vi "DAQ_Static Dig Gen Initialize.vi"(0 "Physical Channels":tag, 7 "Global Channels":refnum<k21>, 11 "error in":errorcluster) -> (4 "DAQmx Task Out":refnum<k21>, 15 "error out":errorcluster)   [LabVIEW 2021, in "DAQ_Static Digital State Generation.lvlib"]
doc: "Initialize Digital Output channels and obtains a DAQmx task\n\nProvide either Physical channel or Global Channel\nIf both physical and Global channels are provided, Global Channels will take precedence\n\n<B>Note:</B> This Library supports only digital line in the physical/global channel. Port is not supported in this library and returns an error. User can either use <B>Dynamic Digital Pattern Measurement Library</B> to support port based inputs or specify the ports in line based format (Ex: <B>DIO/port0/line0:31</B>) with the current library."
uses:
  DAQ_Static Digital State Generation.lvlib
  <vilib>/DAQmx/create/channels.llb/DAQmx Create Channel (DO-Digital Output).vi
panel:
  # "Inputs"
  # "Outputs"
  # "Overview:\nThis VI initializes Digital output channels for static digital generation and provides the DAQmx Task Out\n\nHardware Requirement: A compatible PXI, PCIe, USB, cDAQ or Testscale device\n\nSoftware Requirement: NI DAQmx 2022Q4 or later\n\nInstructions:\n1. Enter physical channel in which Static Digital State Generation has to be done in Physical Channels control. (Or) Enter Global channels to use it instead of initiating a new task. User must configure only one input. If both are provided, Global Channels will take precedence..\n2. Get the Digital Generation task from DAQmx Task Out which stores the reference to the virtual digital output channels.\n\nNotes: \n1. User can use the DAQmx Task on other VI in this library to configure and initiate digital state generation task.\n2. This Library supports only digital line in the physical/global channel. Port is not supported in this library and returns an error. User can either use Dynamic Digital Pattern Measurement Library to support port-based inputs or specify the ports in line based format (Ex: DIO/port0/line0:31) with the current library."
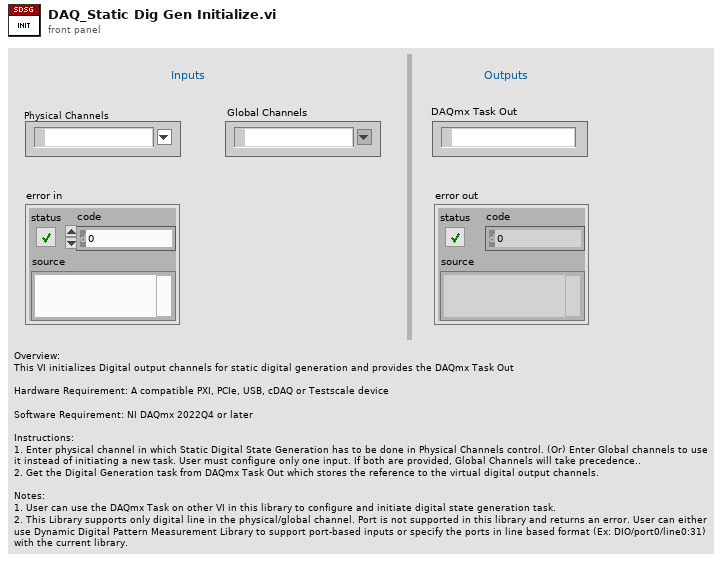
[diagram p1: front panel]
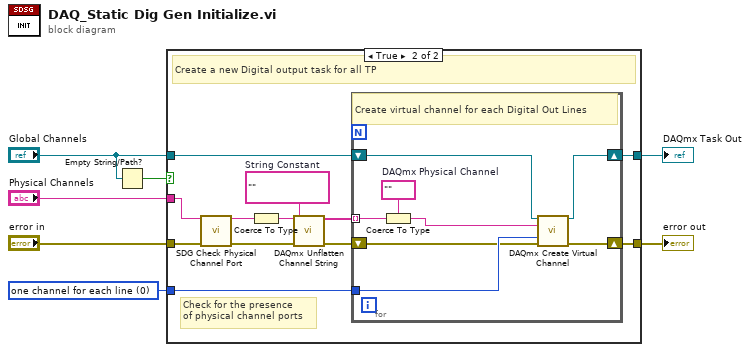
[diagram p0: block diagram]
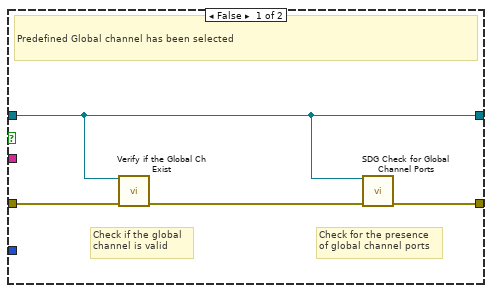
[diagram p2: hidden frame]
diagram:
  w3 = 0 items=["one channel for each line", "one channel for all lines"] ("line grouping")
  n1 = Empty String/Path?(string/path="Global Channels") -> (empty?=w4:bool)
  n2 = case shown="True" w4 {
    tunnel: "Physical Channels" -> [_ w16]
    tunnel: "Global Channels" -> [w11 w23]
    tunnel: [w11 w21] -> w1
    tunnel: "error in" -> [w10 w17]
    tunnel: [w8 w20] -> w2
    tunnel: w3 -> [_ w22]
    frame False {
      # "Check for the presence\nof global channel ports"
      # "Check if the global\nchannel is valid"
      # "Predefined Global channel has been selected"
      n3 = call "Verify if the Global Ch Exist.vi"("Global Channels"=w11, "error in (no error)"=w10) -> ("error out"=w9:errorcluster)  [unwired: 13 in]
      n4 = call "SDG Check for Global Channel Ports.vi"("Global Channel In"=w11, "error in (no error)"=w9) -> ("error out"=w8:errorcluster)  [unwired: 12 in, 1 out]
    }
    frame True {
      w15 = ""  # String Constant
      # "Check for the presence \nof physical channel ports"
      # "Create a new Digital output task for all TP"
      n5 = call "SDG Check Physical Channel Port.vi"("Physical Channel In"=w16, "error in (no error)"=w17) -> ("Physical Channel Out"=w14:tag, "error out"=w12:errorcluster)  [unwired: 12 in]
      n6 = Coerce To Type(0:w14, 1:w15) -> (2:w13:string)
      n7 = call <vilib>:"DAQmx Unflatten Channel String.vi"("names in"=w13, "error in"=w12) -> ("names out"=w19:string[], "error out"=w18:errorcluster)  [unwired: 12 in]
      n8 = for {
        shift-right: [w30] -> w21
        shift-left: w23 -> [w31]
        shift-right: [w29] -> w20
        shift-left: w18 -> [w27]
        tunnel: w19 -> [w26] mode=indexing
        tunnel: w22 -> [w28]
        w25 = tag ""  # DAQmx Physical Channel
        # "Create virtual channel for each Digital Out Lines"
        n9 = Coerce To Type(0:w26, 1:w25) -> (2:w24:tag)
        n10 = call-poly <vilib>:"DAQmx Create Virtual Channel.vi"("task in"=w31, "lines"=w24, "line grouping"=w28, "error in"=w27) -> ("task out"=w30:refnum<k21>, "error out"=w29:errorcluster)  [unwired: 10 in]
      }
    }
  }
  "DAQmx Task Out" <- w1
  "error out" <- w2
